vi "Define Advanced Sequence.vi"(5 "ChannelName":string, 8 "error in (no error)":errorcluster, 10 "Hardware timed Instrument Settings":T1[](array[typedef]) {"SequenceSettings"."Instrument Mode" items=["SMU PS"=1061, "LCR"=1062, "E-Load"=1154]}, 11 "IVI Refnum in":refnum<k15>) -> (0 "error out":errorcluster, 1 "sequence name":string[](array[string]), 3 "IVI Refnum out":refnum<k15>)   [LabVIEW 2023]
uses:
  AdvancedSequenceSettings.ctl
  <instrlib>/niDCPower/nidcpower.llb/niDCPower Sequence Attribute Type.ctl
  <instrlib>/niDCPower/nidcpower.llb/niDCPower Create Advanced Sequence Step With Channels.vi
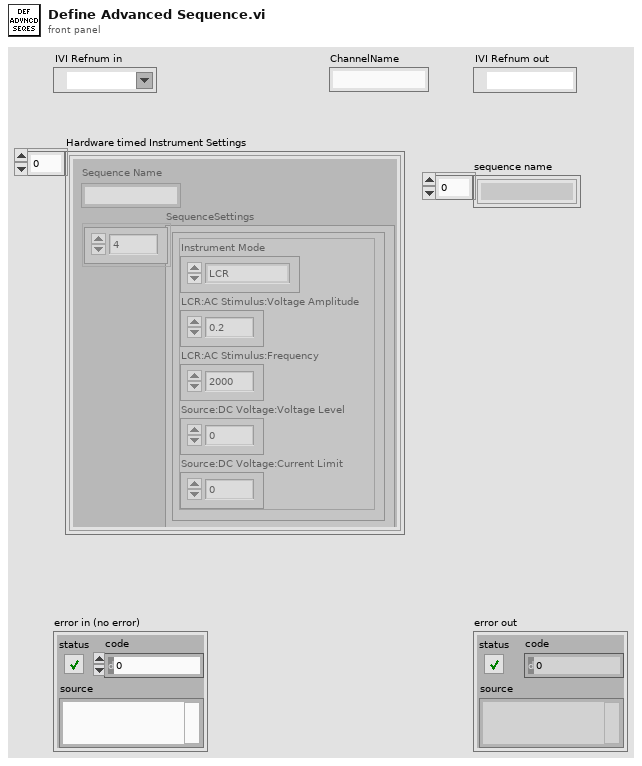
[diagram p1: front panel]
types:
  T1 = typedef "AdvancedSequenceSettings.ctl" = cluster{"Sequence Name":string, "SequenceSettings":cluster{"Instrument Mode":i32, "LCR:AC Stimulus:Voltage Amplitude":dbl, "LCR:AC Stimulus:Frequency":dbl, "Source:DC Voltage:Voltage Level":dbl, "Source:DC Voltage:Current Limit":dbl}[]}
  T2 = typedef "niDCPower Sequence Attribute Type.ctl" = i32
  T3 = cluster{"Instrument Mode":i32, "LCR:AC Stimulus:Voltage Amplitude":dbl, "LCR:AC Stimulus:Frequency":dbl, "Source:DC Voltage:Voltage Level":dbl, "Source:DC Voltage:Current Limit":dbl}[]
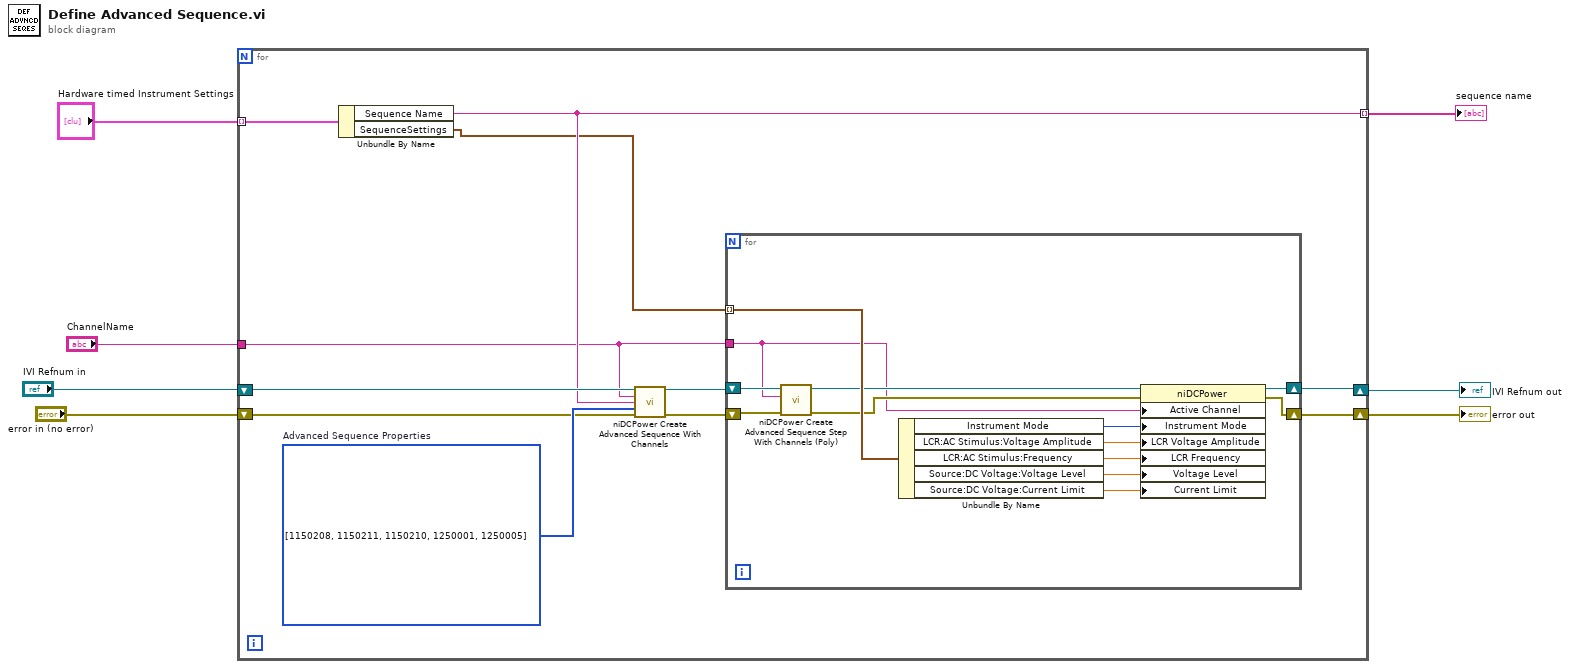
[diagram p0: block diagram]
diagram:
  n1 = for {
    tunnel: "ChannelName" -> [w11]
    tunnel: [w14] -> w4 mode=indexing
    shift-right: [w9] -> w5
    shift-left: "error in (no error)" -> [w17]
    shift-right: [w8] -> w6
    shift-left: "IVI Refnum in" -> [w16]
    tunnel: "Hardware timed Instrument Settings" -> [w15] mode=indexing
    w18 = T2[] [1150208, 1150211, 1150210, 1250001, 1250005] items=["Source -> Output Function"=1150008, "Source -> Output Enabled"=1250006, "Source -> Output Resistance"=1150061, "Source -> Transient Response"=1150062, "Source -> Custom Transient Response -> Voltage Gain Bandwidth"=1150067, "Source -> Custom Transient Response -> Voltage Compensation Frequency"=1150068, "Source -> Custom Transient Response -> Voltage Pole-Zero Ratio"=1150069, "Source -> Custom Transient Response -> Current Gain Bandwidth"=1150070, "Source -> Custom Transient Response -> Current Compensation Frequency"=1150071, "Source -> Custom Transient Response -> Current Pole-Zero Ratio"=1150072, "Source -> DC Voltage -> Voltage Level"=1250001, "Source -> DC Voltage -> Voltage Level Range"=1150005, "Source -> DC Voltage -> Current Limit"=1250005, "Source -> DC Voltage -> Current Limit High"=1150187, "Source -> DC Voltage -> Current Limit Low"=1150188, "Source -> DC Voltage -> Current Limit Range"=1150004, "Source -> DC Current -> Current Level"=1150009, "Source -> DC Current -> Current Level Range"=1150011, "Source -> DC Current -> Voltage Limit"=1150010, "Source -> DC Current -> Voltage Limit High"=1150185, "Source -> DC Current -> Voltage Limit Low"=1150186, "Source -> DC Current -> Voltage Limit Range"=1150012, "Source -> DC Current -> Current Level Slew Rate -> Rising"=1150343, "Source -> DC Current -> Current Level Slew Rate -> Falling"=1150344, "Source -> Pulse Voltage -> Pulse Voltage Level"=1150080, "Source -> Pulse Voltage -> Pulse Bias Voltage Level"=1150082, "Source -> Pulse Voltage -> Pulse Voltage Level Range"=1150084, "Source -> Pulse Voltage -> Pulse Current Limit"=1150081, "Source -> Pulse Voltage -> Pulse Current Limit High"=1150193, "Source -> Pulse Voltage -> Pulse Current Limit Low"=1150194, "Source -> Pulse Voltage -> Pulse Bias Current Limit"=1150083, "Source -> Pulse Voltage -> Pulse Bias Current Limit High"=1150195, "Source -> Pulse Voltage -> Pulse Bias Current Limit Low"=1150196, "Source -> Pulse Voltage -> Pulse Current Limit Range"=1150085, "Source -> Pulse Current -> Pulse Current Level"=1150086, "Source -> Pulse Current -> Pulse Bias Current Level"=1150088, "Source -> Pulse Current -> Pulse Current Level Range"=1150090, "Source -> Pulse Current -> Pulse Voltage Limit"=1150087, "Source -> Pulse Current -> Pulse Voltage Limit High"=1150189, "Source -> Pulse Current -> Pulse Voltage Limit Low"=1150190, "Source -> Pulse Current -> Pulse Bias Voltage Limit"=1150089, "Source -> Pulse Current -> Pulse Bias Voltage Limit High"=1150191, "Source -> Pulse Current -> Pulse Bias Voltage Limit Low"=1150192, "Source -> Pulse Current -> Pulse Voltage Limit Range"=1150091, "Source -> Advanced -> Source Delay"=1150051, "Source -> Advanced -> Pulse Bias Delay"=1150092, "Source -> Advanced -> Pulse On Time"=1150093, "Source -> Advanced -> Pulse Off Time"=1150094, "Source -> Advanced -> OVP Enabled"=1250002, "Source -> Advanced -> OVP Limit"=1250003, "Source -> Advanced -> Compliance Limit Symmetry"=1150184, "Source -> Advanced -> Sequence Step Delta Time"=1150198, "Source -> Advanced -> Conduction Voltage -> Mode"=1150350, "Source -> Advanced -> Conduction Voltage -> On Threshold"=1150351, "Source -> Advanced -> Conduction Voltage -> Off Threshold"=1150352, "Measurement -> Sense"=1150013, "Measurement -> Aperture Time"=1150058, "Measurement -> Measure Record Length"=1150063, "Measurement -> Advanced -> DC Noise Rejection"=1150066, "Measurement -> Autorange"=1150244, "Measurement -> Advanced -> Autorange Behavior"=1150245, "Measurement -> Advanced -> Autorange Aperture Time Mode"=1150246, "Measurement -> Advanced -> Autorange Minimum Aperture Time"=1150247, "Measurement -> Advanced -> Autorange Minimum Aperture Time Units"=1150248, "Measurement -> Advanced -> Autorange Minimum Current Range"=1150255, "Measurement -> Advanced -> Autorange Minimum Voltage Range"=1150256, "Measurement -> Advanced -> Autorange Threshold Mode"=1150257, "Measurement -> Advanced -> Autorange Maximum Delay After Range Change"=1150322, "LCR -> Instrument Mode"=1150208, "LCR -> Source Delay Mode"=1150315, "LCR -> Measurement Time"=1150218, "LCR -> Custom Measurement Time"=1150258, "LCR -> AC Stimulus -> Function"=1150209, "LCR -> AC Stimulus -> Frequency"=1150210, "LCR -> AC Stimulus -> Voltage Amplitude"=1150211, "LCR -> AC Stimulus -> Current Amplitude"=1150212, "LCR -> AC Stimulus -> Advanced -> Voltage Range"=1150265, "LCR -> AC Stimulus -> Advanced -> Current Range"=1150267, "LCR -> AC Stimulus -> Advanced -> Source Aperture Time"=1150349, "LCR -> DC Bias -> Source"=1150213, "LCR -> DC Bias -> Voltage Level"=1150214, "LCR -> DC Bias -> Current Level"=1150215, "LCR -> DC Bias -> Advanced -> Voltage Range"=1150266, "LCR -> DC Bias -> Advanced -> Current Range"=1150274, "LCR -> DC Bias -> Advanced -> Transient Response"=1150347, "LCR -> Compensation -> Open -> Enabled"=1150220, "LCR -> Compensation -> Open -> Conductance"=1150261, "LCR -> Compensation -> Open -> Susceptance"=1150262, "LCR -> Compensation -> Short -> Enabled"=1150221, "LCR -> Compensation -> Short -> Resistance"=1150263, "LCR -> Compensation -> Short -> Reactance"=1150264, "LCR -> Compensation -> Load -> Enabled"=1150222, "LCR -> Compensation -> Load -> Measured Resistance"=1150268, "LCR -> Compensation -> Load -> Measured Reactance"=1150269, "LCR -> Compensation -> Load -> Actual Resistance"=1150270, "LCR -> Compensation -> Load -> Actual Reactance"=1150271, "LCR -> Impedance Range -> Impedance Range"=1150217, "LCR -> Impedance Range -> Impedance Autorange"=1150216, "LCR -> Impedance Range -> Advanced -> Impedance Range Source"=1150321, "LCR -> Impedance Range -> Advanced -> Load Resistance"=1150318, "LCR -> Impedance Range -> Advanced -> Load Inductance"=1150319, "LCR -> Impedance Range -> Advanced -> Load Capacitance"=1150320]  # Advanced Sequence Properties
    n2 = Unbundle By Name(w15) -> ("Sequence Name"=w14:string, "SequenceSettings"=w10:T3)
    n3 = call <instrlib>:"niDCPower Create Advanced Sequence With Channels.vi"("instrument handle"=w16, "channel name"=w11, "sequence name"=w14, "advanced sequence properties"=w18, "error in (no error)"=w17) -> ("instrument handle out"=w13:refnum<k15>, "error out"=w12:errorcluster)  [unwired: 9 in]
    n4 = for {
      tunnel: w11 -> [w19]
      tunnel: w10 -> [w31] mode=indexing
      shift-right: [w29] -> w9
      shift-left: w12 -> [w22]
      shift-right: [w28] -> w8
      shift-left: w13 -> [w23]
      n5 = call-poly <instrlib>:"niDCPower Create Advanced Sequence Step With Channels (Poly).vi"("error in (no error)"=w22, "channel name"=w19, "instrument handle"=w23) -> ("error out"=w21:errorcluster, "instrument handle out"=w20:refnum<k15>)  [unwired: 7 in]
      n6 = Unbundle By Name(w31) -> ("Instrument Mode"=w30:i32, "LCR:AC Stimulus:Voltage Amplitude"=w24:dbl, "LCR:AC Stimulus:Frequency"=w25:dbl, "Source:DC Voltage:Voltage Level"=w27:dbl, "Source:DC Voltage:Current Limit"=w26:dbl)
      n7 = property class="niDCPower"(reference=w20, error in=w21, "Active Channel"=w19, "Instrument Mode"=w30, "LCR Voltage Amplitude"=w24, "LCR Frequency"=w25, "Voltage Level"=w27, "Current Limit"=w26) -> (reference out=w28:refnum<k15>, error out=w29:errorcluster)
    }
  }
  "IVI Refnum out" <- w6
  "error out" <- w5
  "sequence name" <- w4
